vi "PH_Revolver-GUI_6P.calc Position.vi"(1 "Axis Information":T1) -> (0 "Revolver Position":T3 items=["unknown", "Position 0", "Position 60", "Position 120", "Position 180", "Position 240", "Position 300", "moving"])   [LabVIEW 2014, in "PH_Revolver-GUI_6P.lvlib"]
uses:
  PH_Revolver-GUI_6P.lvlib
  PH_Revolver-GUI_6P.Position.ctl
  PH_Basics/PH_Stepmotor_BaseClass/PH_Stepmotor_BaseClass.Axis Information.ctl
  PH_Basics/PH_Stepmotor_BaseClass/PH_Stepmotor_BaseClass.Axis Activity.ctl
  PH_Basics/PH_Stepmotor_BaseClass/PH_Stepmotor_BaseClass.lvlib
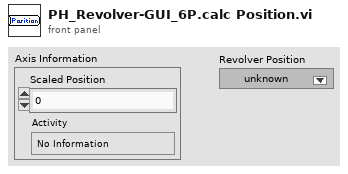
[diagram p1: front panel]
types:
  T1 = typedef "PH_Stepmotor_BaseClass.lvlib/PH_Stepmotor_BaseClass.Axis Information.ctl" = cluster{"Scaled Position":dbl, "Activity":T2}
  T2 = typedef "PH_Stepmotor_BaseClass.lvlib/PH_Stepmotor_BaseClass.Axis Activity.ctl" = enum16{"No Information", "stopped", "running", "Failure", "Alarm", "stopped at backward ES", "stopped at foreward ES"}
  T3 = typedef "PH_Revolver-GUI_6P.lvlib/PH_Revolver-GUI_6P.Position.ctl" = u16
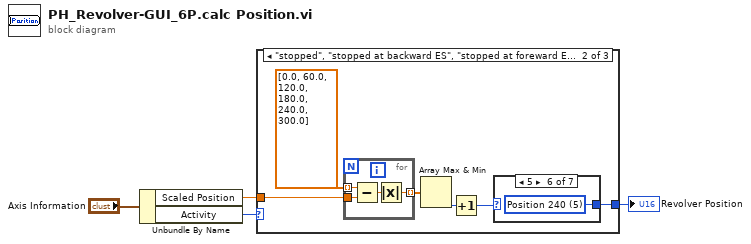
[diagram p0: block diagram]
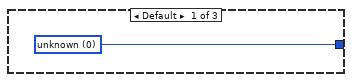
[diagram p2: hidden frame]
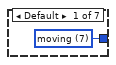
[diagram p3: hidden frame]
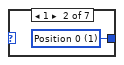
[diagram p4: hidden frame]
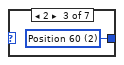
[diagram p5: hidden frame]
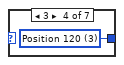
[diagram p6: hidden frame]
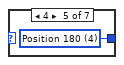
[diagram p7: hidden frame]
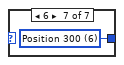
[diagram p8: hidden frame]
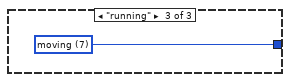
[diagram p9: hidden frame]
diagram:
  n1 = Unbundle By Name("Axis Information") -> ("Scaled Position"=w1:dbl, "Activity"=w3:T2)
  n2 = case shown="\"stopped\", \"stopped at backward ES\", \"stopped at foreward ES\"" w3 {
    tunnel: [w5 w6 w23] -> w2
    tunnel: w1 -> [_ w7 _]
    frame Default {
      w5 = T3 0 items=["unknown", "Position 0", "Position 60", "Position 120", "Position 180", "Position 240", "Position 300", "moving"] ("Revolver Position")
    }
    frame "stopped", "stopped at backward ES", "stopped at foreward ES" {
      n3 = for {
        tunnel: dbl[] [0.0, 60.0, 120.0, 180.0, 240.0, 300.0] -> [w21] mode=indexing
        tunnel: [w19] -> w9 mode=indexing
        tunnel: w7 -> [w20]
        n4 = Subtract(x=w21, y=w20) -> (x-y=w22:dbl)
        n5 = Absolute Value(x=w22) -> (abs(x)=w19:dbl)
      }
      n6 = Array Max & Min(array=w9) -> (min index (indices)=w10:i32)  [unwired: 3 out]
      n7 = Increment(x=w10) -> (x+1=w8:i32)
      n8 = case shown="5" w8 {
        tunnel: [w12 w13 w14 w15 w16 w17 w18] -> w6
        frame Default {
          w12 = T3 7 items=["unknown", "Position 0", "Position 60", "Position 120", "Position 180", "Position 240", "Position 300", "moving"] ("Revolver Position")
        }
        frame 1 {
          w13 = T3 1 items=["unknown", "Position 0", "Position 60", "Position 120", "Position 180", "Position 240", "Position 300", "moving"] ("Revolver Position")
        }
        frame 2 {
          w14 = T3 2 items=["unknown", "Position 0", "Position 60", "Position 120", "Position 180", "Position 240", "Position 300", "moving"] ("Revolver Position")
        }
        frame 3 {
          w15 = T3 3 items=["unknown", "Position 0", "Position 60", "Position 120", "Position 180", "Position 240", "Position 300", "moving"] ("Revolver Position")
        }
        frame 4 {
          w16 = T3 4 items=["unknown", "Position 0", "Position 60", "Position 120", "Position 180", "Position 240", "Position 300", "moving"] ("Revolver Position")
        }
        frame 5 {
          w17 = T3 5 items=["unknown", "Position 0", "Position 60", "Position 120", "Position 180", "Position 240", "Position 300", "moving"] ("Revolver Position")
        }
        frame 6 {
          w18 = T3 6 items=["unknown", "Position 0", "Position 60", "Position 120", "Position 180", "Position 240", "Position 300", "moving"] ("Revolver Position")
        }
      }
    }
    frame "running" {
      w23 = T3 7 items=["unknown", "Position 0", "Position 60", "Position 120", "Position 180", "Position 240", "Position 300", "moving"] ("Revolver Position")
    }
  }
  "Revolver Position" <- w2
